vi "CRYSymbol Conversion.vi"(4 "pGraph VI":refnum<vi>, 6 "CurLib Tab Type":enum16{"Curves", "Values", "Results", "WFM"}(ring), 8 "bData":bool, 9 "nDatas":i32[](array[numeric]), 10 "sData":string, 11 "sActin":string) -> ()   [LabVIEW 2013]
uses:
  Global/CRYCurve Library Global.vi
panel:
  in  "Selected Rows":i32[](array[numeric])
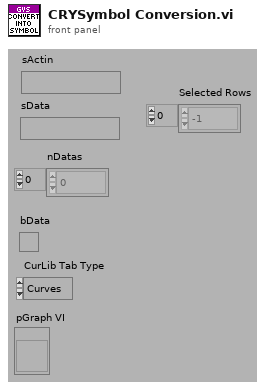
[diagram p1: front panel]
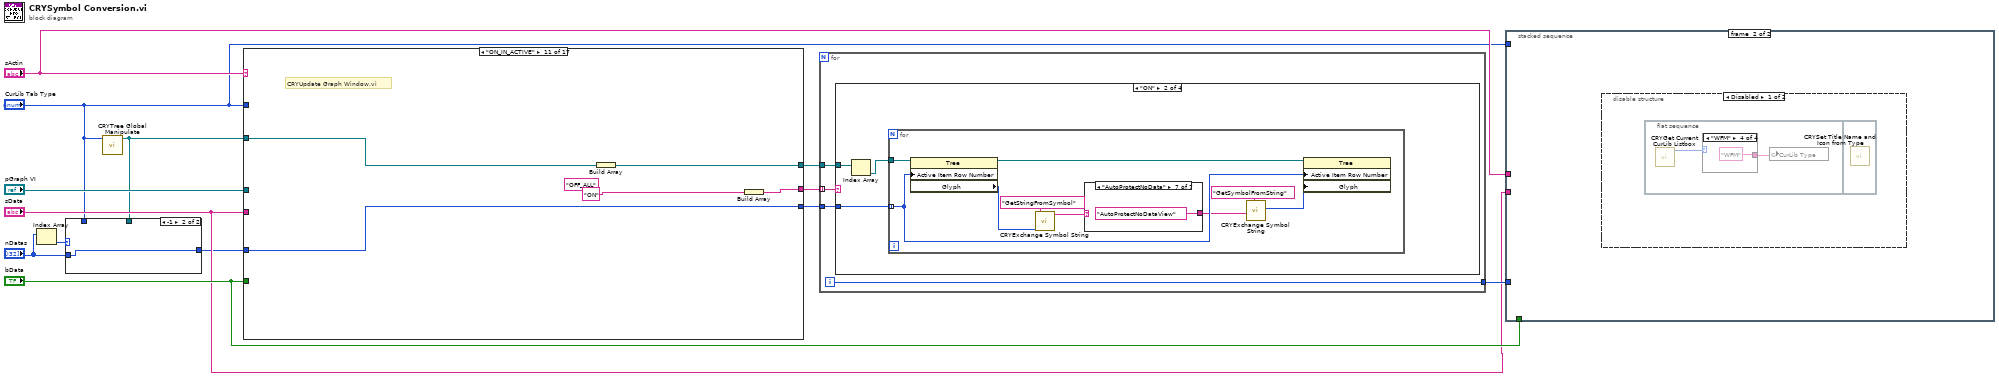
[diagram p0: block diagram]
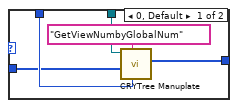
[diagram p2: hidden frame]
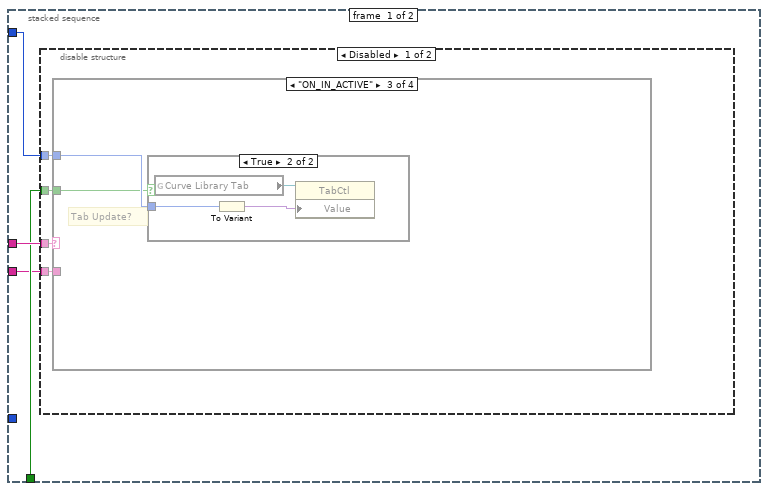
[diagram p3: hidden frame]
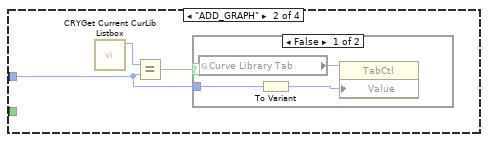
[diagram p5: hidden frame]
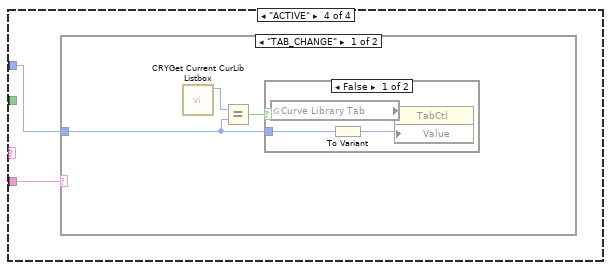
[diagram p8: hidden frame]
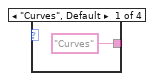
[diagram p12: hidden frame]
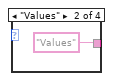
[diagram p13: hidden frame]
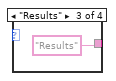
[diagram p14: hidden frame]
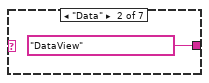
[diagram p18: hidden frame]
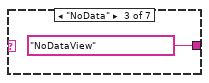
[diagram p19: hidden frame]
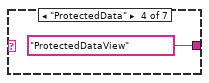
[diagram p20: hidden frame]
diagram:
  n1 = Index Array(array="nDatas") -> (element=w1:i32)  [unwired: 1 in]
  n2 = call "CRYTree Global Manipulate.vi"("Type In"="CurLib Tab Type") -> ("Tree/Curve Tree"=w5:refnum<vi>)  [unwired: 7 in, 3 out]
  n3 = case shown="-1" w1 {
    tunnel: w5 -> [w18 _]
    tunnel: [w17 w19] -> w4
    tunnel: "CurLib Tab Type" -> [w15 _]
    tunnel: "nDatas" -> [w14 w19]
    frame 0, Default {
      n4 = call "CRYTree Manuplate.vi"("Type"=w15, "sAction"="GetViewNumbyGlobalNum", "nData"=w14, "Tree in"=w18) -> ("nData Out"=w17:i32[])  [unwired: 4 in, 3 out]
    }
    frame -1 {
    }
  }
  n5 = case shown="\"ON_IN_ACTIVE\"" "sActin" {
    tunnel: "sData" -> [w21 _ _ _ _ _ _ _ _ _ _ w157 _ _ _ _ _]
    tunnel: w4 -> [w23 w70 w75 w80 w88 _ _ _ _ w146 w152 w158 _ _ w195 _ _]
    tunnel: "CurLib Tab Type" -> [w24 _ _ _ _ w95 w120 _ _ _ _ w154 _ _ _ _ _]
    tunnel: w5 -> [w25 _ _ _ _ _ w124 _ _ _ w151 w156 _ _ w194 _ _]
    tunnel: [w26 w69 w74 w79 w83 w100 w123 w135 w140 w147 w153 w162 refnum<vi>[] [] w188 w193 w200 refnum<vi>[] []] -> w13
    tunnel: [w27 w70 w75 w80 w88 i32[] [] ("nDatas") i32[] [] ("nDatas") i32[] [] ("nDatas") i32[] [] ("nDatas") w146 w152 w158 i32[] [] ("nDatas") w178 w195 i32[] [] ("nDatas") i32[] []] -> w10
    tunnel: [w20 w67 w72 w77 w82 w97 w125 w136 w141 w144 w149 w159 string[] [] w186 w191 w198 w234] -> w12
    tunnel: "bData" -> [_ _ _ _ w87 w96 _ _ _ _ _ _ _ _ _ w201 _]
    tunnel: "pGraph VI" -> [w22 _ _ _ _ _ _ _ _ _ _ _ _ _ _ w199 _]
    frame "LEGEND_REMOVE" {
      n6 = case shown="Default" w21 {
        tunnel: [_ w54] -> w27
        tunnel: [w30 w52] -> w26
        tunnel: [w28 w35] -> w20
        tunnel: w25 -> [_ w50]
        tunnel: w24 -> [_ w49]
        tunnel: w23 -> [_ w47]
        tunnel: w22 -> [_ w40]
        frame "All" {
          n7 = call "CRYTree Global Manipulate.vi"("sOption"="All") -> ("Results Tree"=w31:refnum<vi>, "Values Tree"=w32:refnum<vi>, "Tree/Curve Tree"=w33:refnum<vi>)  [unwired: 7 in, 1 out]
          n8 = Build Array(w33, w32, w31) -> (w30:refnum<vi>[])
          n9 = Build Array("OFF_ALL") -> (w28:string[])
        }
        frame Default {
          n10 = invoke class="VI" method="Ctrl Val.Get"(reference=w40, "Control Name"="GraphType") -> ("Get Control Value Variant"=w46:variant)  [unwired: 2 in, 3 out]
          n11 = invoke class="VI" method="Ctrl Val.Get"(reference=w40, "Control Name"="Legend Ref") -> ("Get Control Value Variant"=w42:variant)  [unwired: 2 in, 3 out]
          n12 = Variant To Data(type="", Variant=w46) -> (data=w36:string)  [unwired: 1 in, 1 out]
          n13 = Variant To Data(type=refnum<vi> refnum ("GMListbox"), Variant=w42) -> (data=w37:refnum<vi>)  [unwired: 1 in, 1 out]
          n14 = call "CRYGet Graph Name From Graph Type.vi"("Graph Type"=w36) -> ("Type"=w48:enum16{"Curves", "Values", "Results", "WFM"})  [unwired: 9 in, 1 out]
          n15 = case shown="Default" w36 {
            tunnel: w50 -> [_ w57]
            tunnel: w49 -> [_ w58]
            tunnel: w48 -> [w56 _]
            tunnel: [w56 w58] -> w38
            tunnel: [w55 w57] -> w39
            frame Default {
              n16 = call "CRYTree Global Manipulate.vi"("Type In"=w56) -> ("Tree/Curve Tree"=w55:refnum<vi>)  [unwired: 7 in, 3 out]
            }
            frame "TABLE" {
            }
          }
          n17 = Index Array(array=w47) -> (element=w53:i32)  [unwired: 1 in]
          n18 = case shown="-1" w53 {
            tunnel: [w59 w64] -> w54
            tunnel: w47 -> [w59 _]
            tunnel: w39 -> [_ w65]
            tunnel: w38 -> [_ w61]
            tunnel: w37 -> [_ w60]
            frame 0, Default {
            }
            frame -1 {
              n19 = call "CRYData View Legend Manipulate.vi"("Type"=w61, "sAction"="GetGlobalNuminLeg", "Legend Ref"=w60) -> ("nData Out"=w62:i32[])  [unwired: 7 in, 1 out]
              n20 = call "CRYTree Manuplate.vi"("Type"=w61, "sAction"="GetViewNumbyGlobalNum", "nData"=w62, "Tree in"=w65) -> ("nData Out"=w64:i32[])  [unwired: 4 in, 3 out]
            }
          }
          n21 = Build Array(w39) -> (w52:refnum<vi>[])
          n22 = Build Array("OFF") -> (w35:string[])
        }
      }
    }
    frame "ON_BY_PLOT" {
      n23 = call "CRYGet Current CurLib Listbox.vi"() -> ("CurLib Tree"=w71:refnum<vi>)  [unwired: 9 in, 2 out]
      n24 = Build Array(w71) -> (w69:refnum<vi>[])
      n25 = Build Array("ON") -> (w67:string[])
    }
    frame "APPEND" {
      n26 = call "CRYGet Current CurLib Listbox.vi"() -> ("CurLib Tree"=w76:refnum<vi>)  [unwired: 9 in, 2 out]
      n27 = Build Array(w76) -> (w74:refnum<vi>[])
      n28 = Build Array("ON") -> (w72:string[])
    }
    frame "SUBTRACT" {
      n29 = call "CRYGet Current CurLib Listbox.vi"() -> ("CurLib Tree"=w81:refnum<vi>)  [unwired: 9 in, 2 out]
      n30 = Build Array(w81) -> (w79:refnum<vi>[])
      n31 = Build Array("OFF") -> (w77:string[])
    }
    frame "ON_IN_PLOT" {
      # "Plot Visible ?"
      n32 = call "CRYGet Current CurLib Listbox.vi"() -> ("CurLib Tree"=w89:refnum<vi>)  [unwired: 9 in, 2 out]
      n33 = Select(t="ON", s=w87, f="OFF") -> (s? t:f=w84:string)
      n34 = Build Array(w89) -> (w83:refnum<vi>[])
      n35 = Build Array(w84) -> (w82:string[])
    }
    frame "OFF_IN_INACTIVE" {
      n36 = call "CRYTree Global Manipulate.vi"("sOption"="All") -> ("WFM Tree"=w90:refnum<vi>, "Results Tree"=w91:refnum<vi>, "Values Tree"=w92:refnum<vi>, "Tree/Curve Tree"=w93:refnum<vi>)  [unwired: 7 in]
      n37 = case shown="\"Curves\", Default" w95 {
        tunnel: [w107 w111 w115 w119] -> w100
        tunnel: w93 -> [_ w110 w114 w118]
        tunnel: w92 -> [w106 _ w113 w117]
        tunnel: w91 -> [w105 w109 _ w116]
        tunnel: w90 -> [w104 w108 w112 _]
        frame "Curves", Default {
          n38 = Build Array(w106, w105, w104) -> (w107:refnum<vi>[])
        }
        frame "Values" {
          n39 = Build Array(w110, w109, w108) -> (w111:refnum<vi>[])
        }
        frame "Results" {
          n40 = Build Array(w114, w113, w112) -> (w115:refnum<vi>[])
        }
        frame "WFM" {
          n41 = Build Array(w118, w117, w116) -> (w119:refnum<vi>[])
        }
      }
      n42 = case shown="True" w96 {
        tunnel: w95 -> [_ w102]
        frame False {
        }
        frame True {
          n43 = global read "CRYCurve Library Global.vi" "Curve Library Tab"() -> (w103:refnum<vi>)
          n44 = To Variant(anything=w102) -> (Variant=w101:variant)
          n45 = property class="TabCtl"(reference=w103, "Value"=w101) -> ()  [unwired: 1 in, 2 out]
        }
      }
      n46 = Build Array("OFF_ALL") -> (w97:string[])
    }
    frame "ADD_GRAPH" {
      n47 = call "CRYGet Current CurLib Listbox.vi"() -> ("Type"=w121:enum16{"Curves", "Values", "Results", "WFM"})  [unwired: 9 in, 2 out]
      n48 = Equal?(x=w121, y=w120) -> (x = y?=w122:bool)
      n49 = case shown="False" w122 {
        tunnel: w120 -> [w129 _]
        frame False {
          n50 = global read "CRYCurve Library Global.vi" "Curve Library Tab"() -> (w130:refnum<vi>)
          n51 = To Variant(anything=w129) -> (Variant=w128:variant)
          n52 = property class="TabCtl"(reference=w130, "Value"=w128) -> ()  [unwired: 1 in, 2 out]
        }
        frame True {
        }
      }
      n53 = Build Array("OFF_ALL") -> (w125:string[])
      n54 = Build Array(w124) -> (w123:refnum<vi>[])
    }
    frame "VIEW_CLOSE" {
      n55 = call "CRYTree Global Manipulate.vi"("sOption"="All") -> ("Results Tree"=w131:refnum<vi>, "Values Tree"=w132:refnum<vi>, "Tree/Curve Tree"=w133:refnum<vi>)  [unwired: 7 in, 1 out]
      n56 = Build Array(w133, w132, w131) -> (w135:refnum<vi>[])
      n57 = Build Array("OFF_ALL") -> (w136:string[])
    }
    frame "CURLIB_CLICK" {
      n58 = call "CRYGet Current CurLib Listbox.vi"() -> ("CurLib Tree"=w139:refnum<vi>)  [unwired: 9 in, 2 out]
      n59 = Build Array("OFF_ALL") -> (w141:string[])
      n60 = Build Array(w139) -> (w140:refnum<vi>[])
    }
    frame "ON_IN_GRAPH CLICKING" {
      n61 = call "CRYGet Current CurLib Listbox.vi"() -> ("CurLib Tree"=w148:refnum<vi>)  [unwired: 9 in, 2 out]
      n62 = Build Array("ON") -> (w144:string[])
      n63 = Build Array(w148) -> (w147:refnum<vi>[])
    }
    frame "ON_IN_ACTIVE" {
      (unwired) "OFF_ALL"
      # "CRYUpdate Graph Window.vi"
      n64 = Build Array(w151) -> (w153:refnum<vi>[])
      n65 = Build Array("ON") -> (w149:string[])
    }
    frame "ACTIVE" {
      n66 = case shown="\"TAB_CHANGE\"" w157 {
        tunnel: w156 -> [w166 _]
        tunnel: [w166 w170] -> w155
        tunnel: w154 -> [w163 _]
        frame "TAB_CHANGE" {
          n67 = call "CRYGet Current CurLib Listbox.vi"() -> ("Type"=w164:enum16{"Curves", "Values", "Results", "WFM"})  [unwired: 9 in, 2 out]
          n68 = Equal?(x=w164, y=w163) -> (x = y?=w165:bool)
          n69 = case shown="True" w165 {
            tunnel: w163 -> [w168 _]
            frame False {
              n70 = global read "CRYCurve Library Global.vi" "Curve Library Tab"() -> (w169:refnum<vi>)
              n71 = To Variant(anything=w168) -> (Variant=w167:variant)
              n72 = property class="TabCtl"(reference=w169, "Value"=w167) -> ()  [unwired: 1 in, 2 out]
            }
            frame True {
            }
          }
        }
        frame "TAB_NOCHANGE", Default {
          n73 = call "CRYGet Current CurLib Listbox.vi"() -> ("CurLib Tree"=w170:refnum<vi>)  [unwired: 9 in, 2 out]
        }
      }
      n74 = Build Array(w155) -> (w162:refnum<vi>[])
      n75 = Build Array("OFF_ALL", "ON") -> (w159:string[])
    }
    frame "NONE" {
    }
    frame "ON_BY_POPUP" {
      n76 = call "CRYGet Current CurLib Listbox.vi"() -> ("CurLib Tree"=w177:refnum<vi>)  [unwired: 9 in, 2 out]
      n77 = call "CRYTree Manuplate.vi"("sAction"="GetActiveNumbers", "Tree in"=w177) -> ("nData Out"=w175:i32[], "Tree Out"=w174:refnum<vi>)  [unwired: 6 in, 2 out]
      n78 = Array Size(array="Selected Rows") -> (size(s)=w181:i32)
      n79 = Array Size(array=w175) -> (size(s)=w183:i32)
      n80 = Equal To 0?(x=w181) -> (x = 0?=w179:bool)
      n81 = Greater Or Equal?(x=w183, y=2) -> (x >= y?=w180:bool)
      n82 = Or(x=w180, y=w179) -> (x .or. y?=w184:bool)
      n83 = case shown="False" w184 {
        tunnel: [w189 w190] -> w178
        tunnel: w175 -> [_ w190]
        tunnel: "Selected Rows" -> [w189 _]
        frame False {
        }
        frame True {
        }
      }
      n84 = Build Array("ON") -> (w186:string[])
      n85 = Build Array(w174) -> (w188:refnum<vi>[])
    }
    frame "ON_BY_UPDATE" {
      n86 = Build Array(w194) -> (w193:refnum<vi>[])
      n87 = Build Array("ON") -> (w191:string[])
    }
    frame "OFF_IN_REMOVE" {
      # "One/All"
      n88 = Not A Number/Path/Refnum?(number/path/refnum=w199) -> (NaN/Path/Refnum?=w197:bool)
      n89 = case shown="True" w197 {
        tunnel: w201 -> [_ w208]
        tunnel: [refnum<vi>[] [] w207] -> w200
        tunnel: w199 -> [_ w206]
        tunnel: [string[] [] w204] -> w198
        frame False {
        }
        frame True {
          n90 = case shown="True" w208 {
            tunnel: [w218 w233] -> w207
            tunnel: w206 -> [w214 _]
            frame False {
              n91 = invoke class="VI" method="Ctrl Val.Get"(reference=w214, "Control Name"="GraphType") -> ("Get Control Value Variant"=w215:variant)  [unwired: 2 in, 3 out]
              n92 = Variant To Data(type="", Variant=w215) -> (data=w213:string)  [unwired: 1 in, 1 out]
              n93 = call "CRYTree Global Manipulate.vi"() -> ("WFM Tree"=w209:refnum<vi>, "Results Tree"=w210:refnum<vi>, "Values Tree"=w211:refnum<vi>, "Tree/Curve Tree"=w212:refnum<vi>)  [unwired: 8 in]
              n94 = case shown="\"BAR\", \"DIGITAL\", \"POLAR\", \"XY\", Default" w213 {
                tunnel: [w220 w223 w225 w227] -> w218
                tunnel: w212 -> [w219 w222 _ _]
                tunnel: w211 -> [_ w221 _ _]
                tunnel: w210 -> [_ _ w224 _]
                tunnel: w209 -> [_ _ _ w226]
                frame "BAR", "DIGITAL", "POLAR", "XY", Default {
                  n95 = Build Array(w219) -> (w220:refnum<vi>[])
                }
                frame "TABLE" {
                  n96 = Build Array(w222, w221) -> (w223:refnum<vi>[])
                }
                frame "RESULT" {
                  n97 = Build Array(w224) -> (w225:refnum<vi>[])
                }
                frame "WAVE" {
                  n98 = Build Array(w226) -> (w227:refnum<vi>[])
                }
              }
            }
            frame True {
              n99 = call "CRYTree Global Manipulate.vi"("sOption"="All") -> ("WFM Tree"=w228:refnum<vi>, "Results Tree"=w229:refnum<vi>, "Values Tree"=w230:refnum<vi>, "Tree/Curve Tree"=w231:refnum<vi>)  [unwired: 7 in]
              n100 = Build Array(w231, w230, w229, w228) -> (w233:refnum<vi>[])
            }
          }
          n101 = Build Array("OFF_ALL") -> (w204:string[])
        }
      }
    }
    frame Default {
      n102 = Build Array("") -> (w234:string[])
    }
  }
  n103 = for {
    tunnel: w13 -> [w241]
    tunnel: w10 -> [w240]
    tunnel: w12 -> [w239] mode=indexing
    tunnel: [w238] -> w8
    i -> [w238]
    n104 = case shown="\"ON\"" w239 {
      tunnel: w241 -> [_ w243 w262 w280]
      tunnel: w240 -> [_ w244 w263 _]
      frame Default {
      }
      frame "ON" {
        n105 = Index Array(array=w243) -> (element=w242:refnum<vi>)  [unwired: 1 in]
        n106 = for {
          tunnel: w242 -> [w253]
          tunnel: w244 -> [w251] mode=indexing
          n107 = property on="Property Node" class="Tree"(reference=w253, "Active Item Row Number"=w251) -> (reference out=w252:refnum<vi>, "Glyph"=w248:i32)  [unwired: 1 in, 1 out]
          n108 = call "CRYExchange Symbol String.vi"("nData"=w248, "sAction"="GetStringFromSymbol") -> ("sData out"=w249:string)  [unwired: 8 in, 1 out]
          n109 = case shown="\"AutoProtectNoData\"" w249 {
            selector: w249 -> [w254 _ _ _ _ _ _]
            tunnel: [w254 "DataView" ("name or relative path") "NoDataView" ("name or relative path") "ProtectedDataView" ("name or relative path") "ProtectedNoDataView" ("name or relative path") "AutoProtectDataView" ("name or relative path") "AutoProtectNoDataView" ("name or relative path")] -> w246
            frame Default {
            }
            frame "Data" {
            }
            frame "NoData" {
            }
            frame "ProtectedData" {
            }
            frame "ProtectedNoData" {
            }
            frame "AutoProtectData" {
            }
            frame "AutoProtectNoData" {
            }
          }
          n110 = call "CRYExchange Symbol String.vi"("sData"=w246, "sAction"="GetSymbolFromString") -> ("nData out"=w245:i32)  [unwired: 8 in, 1 out]
          n111 = property on="Property Node" class="Tree"(reference=w252, "Active Item Row Number"=w251, "Glyph"=w245) -> ()  [unwired: 1 in, 2 out]
        }
      }
      frame "OFF" {
        n112 = Index Array(array=w262) -> (element=w261:refnum<vi>)  [unwired: 1 in]
        n113 = for {
          tunnel: w261 -> [w272]
          tunnel: w263 -> [w270] mode=indexing
          n114 = property on="Property Node" class="Tree"(reference=w272, "Active Item Row Number"=w270) -> (reference out=w271:refnum<vi>, "Glyph"=w268:i32)  [unwired: 1 in, 1 out]
          n115 = call "CRYExchange Symbol String.vi"("nData"=w268, "sAction"="GetStringFromSymbol") -> ("sData out"=w267:string)  [unwired: 8 in, 1 out]
          n116 = case shown="\"AutoProtectNoDataView\"" w267 {
            selector: w267 -> [w273 _ _ _ _ _ _]
            tunnel: [w273 "Data" ("name or relative path") "NoData" ("name or relative path") "ProtectedData" ("name or relative path") "ProtectedNoData" ("name or relative path") "AutoProtectData" ("name or relative path") "AutoProtectNoData" ("name or relative path")] -> w264
            frame Default {
            }
            frame "DataView" {
            }
            frame "NoDataView" {
            }
            frame "ProtectedDataView" {
            }
            frame "ProtectedNoDataView" {
            }
            frame "AutoProtectDataView" {
            }
            frame "AutoProtectNoDataView" {
            }
          }
          n117 = call "CRYExchange Symbol String.vi"("sData"=w264, "sAction"="GetSymbolFromString") -> ("nData out"=w265:i32)  [unwired: 8 in, 1 out]
          n118 = property on="Property Node" class="Tree"(reference=w271, "Active Item Row Number"=w270, "Glyph"=w265) -> ()  [unwired: 1 in, 2 out]
        }
      }
      frame "OFF_ALL" {
        n119 = for {
          tunnel: w280 -> [w281] mode=indexing
          n120 = call "CRYTree Manuplate.vi"("sAction"="GetTotalCount", "Tree in"=w281) -> ("nData Out"=w283:i32[])  [unwired: 6 in, 3 out]
          n121 = Index Array(array=w283) -> (element=w282:i32)  [unwired: 1 in]
          n122 = for {
            N: w282 -> [_]
            tunnel: w281 -> [w293]
            i -> [w291]
            n123 = property on="Property Node" class="Tree"(reference=w293, "Active Item Row Number"=w291) -> (reference out=w292:refnum<vi>, "Glyph"=w289:i32)  [unwired: 1 in, 1 out]
            n124 = call "CRYExchange Symbol String.vi"("nData"=w289, "sAction"="GetStringFromSymbol") -> ("sData out"=w288:string)  [unwired: 8 in, 1 out]
            n125 = case shown="Default" w288 {
              selector: w288 -> [w294 _ _ _ _ _ _]
              tunnel: [w294 "Data" ("name or relative path") "NoData" ("name or relative path") "ProtectedData" ("name or relative path") "ProtectedNoData" ("name or relative path") "AutoProtectData" ("name or relative path") "AutoProtectNoData" ("name or relative path")] -> w286
              frame Default {
              }
              frame "DataView" {
              }
              frame "NoDataView" {
              }
              frame "ProtectedDataView" {
              }
              frame "ProtectedNoDataView" {
              }
              frame "AutoProtectDataView" {
              }
              frame "AutoProtectNoDataView" {
              }
            }
            n126 = call "CRYExchange Symbol String.vi"("sData"=w286, "sAction"="GetSymbolFromString") -> ("nData out"=w285:i32)  [unwired: 8 in, 1 out]
            n127 = property on="Property Node" class="Tree"(reference=w292, "Active Item Row Number"=w291, "Glyph"=w285) -> ()  [unwired: 1 in, 2 out]
          }
        }
      }
    }
  }
  n128 = stacked-sequence {
    tunnel: "sActin" -> [w304 _]
    tunnel: w8 -> [_ _]
    tunnel: "CurLib Tab Type" -> [w303 _]
    tunnel: "bData" -> [w302 _]
    tunnel: "sData" -> [w301 _]
    frame #0 {
      n129 = disable-structure shown="Disabled" {
        disable-tunnel: w304 -> [w308 _]
        disable-tunnel: w303 -> [w307 _]
        disable-tunnel: w302 -> [w306 _]
        disable-tunnel: w301 -> [w305 _]
        frame Disabled {
          n130 = case shown="\"ON_IN_ACTIVE\"" w308 {
            tunnel: w307 -> [_ w309 w316 w321]
            tunnel: w306 -> [_ _ w315 _]
            tunnel: w305 -> [_ _ _ w320]
            frame Default {
            }
            frame "ADD_GRAPH" {
              n131 = call "CRYGet Current CurLib Listbox.vi"() -> ("Type"=w310:enum16{"Curves", "Values", "Results", "WFM"})  [unwired: 9 in, 2 out]
              n132 = Equal?(x=w310, y=w309) -> (x = y?=w311:bool)
              n133 = case shown="False" w311 {
                tunnel: w309 -> [w313 _]
                frame False {
                  n134 = global read "CRYCurve Library Global.vi" "Curve Library Tab"() -> (w314:refnum<vi>)
                  n135 = To Variant(anything=w313) -> (Variant=w312:variant)
                  n136 = property class="TabCtl"(reference=w314, "Value"=w312) -> ()  [unwired: 1 in, 2 out]
                }
                frame True {
                }
              }
            }
            frame "ON_IN_ACTIVE" {
              # "Tab Update?"
              n137 = case shown="True" w315 {
                tunnel: w316 -> [_ w318]
                frame False {
                }
                frame True {
                  n138 = global read "CRYCurve Library Global.vi" "Curve Library Tab"() -> (w319:refnum<vi>)
                  n139 = To Variant(anything=w318) -> (Variant=w317:variant)
                  n140 = property class="TabCtl"(reference=w319, "Value"=w317) -> ()  [unwired: 1 in, 2 out]
                }
              }
            }
            frame "ACTIVE" {
              n141 = case shown="\"TAB_CHANGE\"" w320 {
                tunnel: w321 -> [w323 _]
                frame "TAB_CHANGE" {
                  n142 = call "CRYGet Current CurLib Listbox.vi"() -> ("Type"=w324:enum16{"Curves", "Values", "Results", "WFM"})  [unwired: 9 in, 2 out]
                  n143 = Equal?(x=w324, y=w323) -> (x = y?=w322:bool)
                  n144 = case shown="False" w322 {
                    tunnel: w323 -> [w326 _]
                    frame False {
                      n145 = global read "CRYCurve Library Global.vi" "Curve Library Tab"() -> (w327:refnum<vi>)
                      n146 = To Variant(anything=w326) -> (Variant=w325:variant)
                      n147 = property class="TabCtl"(reference=w327, "Value"=w325) -> ()  [unwired: 1 in, 2 out]
                    }
                    frame True {
                    }
                  }
                }
                frame "TAB_NOCHANGE", Default {
                }
              }
            }
          }
        }
        frame Enabled {
        }
      }
    }
    frame #1 {
      n148 = disable-structure shown="Disabled" {
        frame Disabled {
          n149 = flat-sequence {
            frame #0 {
              n150 = call "CRYGet Current CurLib Listbox.vi"() -> ("Type"=w328:enum16{"Curves", "Values", "Results", "WFM"})  [unwired: 9 in, 2 out]
              n151 = case shown="\"WFM\"" w328 {
                tunnel: ["Curves" "Values" "Results" "WFM"] -> w329
                frame "Curves", Default {
                }
                frame "Values" {
                }
                frame "Results" {
                }
                frame "WFM" {
                }
              }
              n152 = global write "CRYCurve Library Global.vi" "CurLib Type"(w329) -> ()
            }
            frame #1 {
              n153 = call "CRYSet Title Name and Icon from Type.vi"() -> ()  [unwired: 12 in]
            }
          }
        }
        frame Enabled {
        }
      }
    }
  }
